vi "SWERVE_TRAJECTORY_READFILE_BEGIN.vi"(8 "ABS Odo Initialize":bool, 9 "Starting ChassisSpeeds":T4 {"vOmega" format="%10.3f"; "vY" format="%10.3f"; "vX" format="%10.3f"}, 10 "Write_Traj":bool=TRUE, 11 "Trajectory File Name":string="Sample-Robot-2-Trajectory-TrajLibrary.csv") -> (0 "error out":errorcluster, 1 "StartingPose":T1={"TRANSLATION"={"X"=0.0, "Y"=0.0}, "ROTATION"={"VALUE"=0.0, "COS"=1.0, "SIN"=0.0}} {"ROTATION"."SIN" format="%13.4f"; "ROTATION"."COS" format="%13.4f"; "ROTATION"."VALUE" format="%13.4f"; "TRANSLATION"."Y" format="%14.3f"; "TRANSLATION"."X" format="%14.3f"}, 2 "Trajectory Items":i32, 3 "TotalTImeSecs":dbl)   [LabVIEW 2023]
uses:
  <vilib>/Rock Robotics/WPI/ThirdParty/JAS_Junk/TrajLib/TypeDef/CHASSIS_SPEEDS.ctl
  <vilib>/Rock Robotics/WPI/ThirdParty/JAS_Junk/TrajLib/TypeDef/POSE2D.ctl
  <vilib>/Rock Robotics/WPI/ThirdParty/JAS_Junk/TrajLib/TypeDef/TRANSLATION2D.ctl
  <vilib>/Rock Robotics/WPI/ThirdParty/JAS_Junk/TrajLib/TypeDef/ROTATION2D.ctl
  <vilib>/Rock Robotics/WPI/ThirdParty/MJansen/PathPlanner/TypeDef/PathPlannerTrajectory.ctl
  <vilib>/Rock Robotics/WPI/ThirdParty/MJansen/PathPlanner/TypeDef/PathPlannerTrajectoryState.ctl
  <vilib>/Rock Robotics/WPI/ThirdParty/MJansen/PathPlanner/TypeDef/PathPlannerPathConstraints.ctl
  <vilib>/Rock Robotics/WPI/ThirdParty/MJansen/PathPlanner/TypeDef/PathPlannerPath.ctl
  <vilib>/Rock Robotics/WPI/ThirdParty/MJansen/PathPlanner/TypeDef/PathPlannerRotationTarget.ctl
  <vilib>/Rock Robotics/WPI/ThirdParty/MJansen/PathPlanner/TypeDef/PathPlannerConstraintsZone.ctl
  <vilib>/Rock Robotics/WPI/ThirdParty/MJansen/PathPlanner/TypeDef/PathPlannerEventMarker.ctl
  <vilib>/Rock Robotics/WPI/ThirdParty/MJansen/PathPlanner/TypeDef/PathPlannerCommandUtil.ctl
  <vilib>/Rock Robotics/WPI/ThirdParty/MJansen/PathPlanner/ENum/PathPlanner_CommandUtilType_ENUM.ctl
  <vilib>/Rock Robotics/WPI/ThirdParty/MJansen/PathPlanner/TypeDef/PathPlannerGoalEndState.ctl
  <vilib>/Rock Robotics/WPI/ThirdParty/MJansen/PathPlanner/TypeDef/PathPlannerPathPoint.ctl
  <vilib>/Rock Robotics/WPI/ThirdParty/MJansen/PathPlanner/VI/PathPlanner_Path_GetPoint.vi
  <vilib>/Rock Robotics/WPI/ThirdParty/JAS_Junk/TrajLib/Pose2d_New_TRRO.vi
  <vilib>/Rock Robotics/WPI/ThirdParty/MJansen/PathPlanner/VI/PathPlanner_PathPoint_GetAll.vi
  <vilib>/Rock Robotics/WPI/ThirdParty/JAS_Junk/TrajLib/Pose2d_getRotation.vi
  <vilib>/Rock Robotics/WPI/ThirdParty/JAS_Junk/TrajLib/Rotation2d_Minus.vi
  <vilib>/Rock Robotics/WPI/ThirdParty/JAS_Junk/TrajLib/VI/TimeInterpVariant_Clear.vi
  <vilib>/Rock Robotics/WPI/ThirdParty/JAS_Junk/TrajLib/Rotation2d_UnaryMinus.vi
  <vilib>/Rock Robotics/WPI/ThirdParty/JAS_Junk/TrajLib/Rotation2d_RotateBy.vi
  <vilib>/Rock Robotics/WPI/ThirdParty/JAS_Junk/TrajLib/Rotation2d_CreateXY.vi
  <vilib>/Rock Robotics/WPI/ThirdParty/JAS_Junk/TrajLib/Util_CalcDist.vi
  Swerve_Drive_System/SWERVE_DRIVE_GLOBALS.vi
  <vilib>/Rock Robotics/WPI/ThirdParty/JAS_Junk/TrajLib/Trajectory_Library.lvlib
  <vilib>/Rock Robotics/WPI/ThirdParty/MJansen/PathPlanner/PathPlanner24.lvlib
panel:
  # "Relative or absolute trajectory\nfile name"
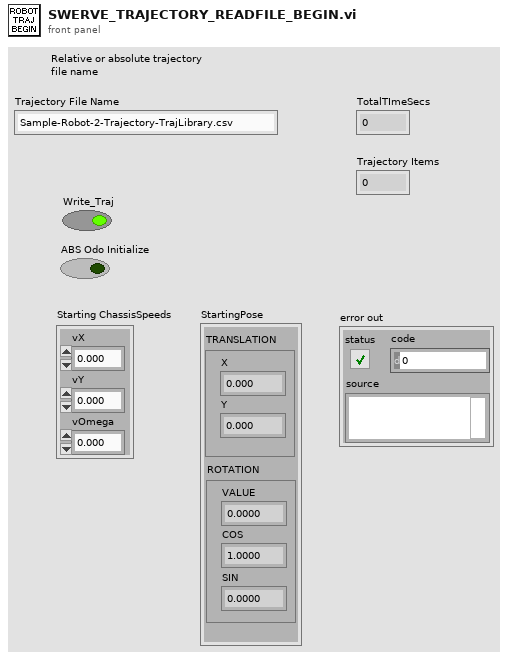
[diagram p1: front panel]
types:
  T1 = typedef "Trajectory_Library.lvlib/POSE2D.ctl" = cluster{"TRANSLATION":T2, "ROTATION":T3}
  T2 = typedef "Trajectory_Library.lvlib/TRANSLATION2D.ctl" = cluster{"X":dbl, "Y":dbl}
  T3 = typedef "Trajectory_Library.lvlib/ROTATION2D.ctl" = cluster{"VALUE":dbl, "COS":dbl, "SIN":dbl}
  T4 = typedef "Trajectory_Library.lvlib/CHASSIS_SPEEDS.ctl" = cluster{"vX":dbl, "vY":dbl, "vOmega":dbl}
  T5 = typedef "PathPlanner24.lvlib/PathPlannerPath.ctl" = cluster{"BezierPoints":T2[], "PreviewStartingRotation":T3, "Reversed":bool, "RotationTargets":T6[], "ConstraintZones":T7[], "EventMarkers":T9[], "GlobalConstraints":T8, "GoalEndState":T12, "AllPoints":T13[]}
  T6 = typedef "PathPlanner24.lvlib/PathPlannerRotationTarget.ctl" = cluster{"target":T3, "WaypointRelativePosition":dbl, "Exists":bool}
  T7 = typedef "PathPlanner24.lvlib/PathPlannerConstraintsZone.ctl" = cluster{"minWaypointPos":dbl, "maxWaypointPos":dbl, "Constraints":T8, "Present":bool}
  T8 = typedef "PathPlanner24.lvlib/PathPlannerPathConstraints.ctl" = cluster{"MaxVelocityMps;":dbl, "MaxAccelerationMpsSq;":dbl, "MaxAngularVelRadPsEc;":dbl, "MaxAngularAccRadPSecSq":dbl, "Exists":bool}
  T9 = typedef "PathPlanner24.lvlib/PathPlannerEventMarker.ctl" = cluster{"WaypointRelativePos":dbl, "minimumTriggerDistance":dbl, "markerPos":T2, "lastRobotPos":T2, "Command":T10, "markerPos Exists":bool, "LastRobotPoseExists":bool, "Triggered":bool}
  T10 = typedef "PathPlanner24.lvlib/PathPlannerCommandUtil.ctl" = cluster{"waitTime":dbl, "name":string, "pathName":string, "commands":cluster{"type":T11, "waitTime":dbl, "name":string, "pathName":string}[], "type":T11}
  T11 = typedef "PathPlanner24.lvlib/PathPlanner_CommandUtilType_ENUM.ctl" = enum16{"Unknown", "Wait", "Named", "Path", "Sequential", "Parallel", "Race", "Deadline"}
  T12 = typedef "PathPlanner24.lvlib/PathPlannerGoalEndState.ctl" = cluster{"Velocity":dbl, "Rotation":T3}
  T13 = typedef "PathPlanner24.lvlib/PathPlannerPathPoint.ctl" = cluster{"Position":T2, "HolonomicRotation":T3, "DistAlongPath":dbl, "CurveRadius":dbl, "MaxV":dbl, "Constraints":T8, "HolonomicRotationExists":bool}
  T14 = typedef "PathPlanner24.lvlib/PathPlannerTrajectory.ctl" = cluster{"States":T15[]}
  T15 = typedef "PathPlanner24.lvlib/PathPlannerTrajectoryState.ctl" = cluster{"TimeSeconds":dbl, "VelocityMPS":dbl, "AccerationMpsSq":dbl, "HeadingAngularVelRadPerSec":dbl, "PositionMeters":T2, "Heading":T3, "TargetHolonomicRotation":T3, "CurvatureRadPerMeter":dbl, "PathPlannerConstraints":T8, "DeltaPos":dbl}
  T16 = typedef "Trajectory_Library.lvlib/TRAJECTORY.ctl" = cluster{"TotalTImeSecs":dbl, "States":T17[]}
  T17 = typedef "Trajectory_Library.lvlib/TRAJ_STATE.ctl" = cluster{"TimeSeconds":dbl, "Velocity":dbl, "Acceleration":dbl, "POSE":T1, "Curvature":dbl}
  T18 = typedef "Trajectory_Library.lvlib/SWERVE_DRIVE_POSE_EST2.ctl" = cluster{"M_Vision_K":T19, "m_nominal_dT":dbl, "m_PrevTime_Sec":dbl, "Pose_Buffer":T20, "Swerve_Drive_Kinematics":T21, "Swerve_Drive_Odom":T23, "M_Q":T19, "NumModules":i32}
  T19 = typedef "NI_Matrix.lvlib/RealMatrix.ctl" = dbl[][]
  T20 = typedef "Trajectory_Library.lvlib/TIME_INTERPOLATABLE_VARIANT.ctl" = cluster{"TimeStamps":dbl[], "DataArray":variant[], "Min_TimeStamp":dbl, "Max_TimeStamp":dbl, "ItemCount":i32, "MaxBufferTime":dbl}
  T21 = typedef "Trajectory_Library.lvlib/SWERVE_DRIVE_KINEMATICS.ctl" = cluster{"NumModules":i32, "InverseKinematics":T19, "ForwardKinematics":T19, "Modules":T2[], "PrevCoR":T2, "SavedModuleStates":T22[]}
  T22 = typedef "Trajectory_Library.lvlib/SWERVE_DRIVE_MODULE_STATE.ctl" = cluster{"Speed":dbl, "Angle":T3}
  T23 = typedef "Trajectory_Library.lvlib/SWERVE_DRIVE_ODOMETRY.ctl" = cluster{"POSE":T1, "GyroOffset":T3, "PreviousAngle":T3, "PrevModulePositions":T24[], "NumModules":i32}
  T24 = typedef "Trajectory_Library.lvlib/SWERVE_DRIVE_MODULE_POSITION.ctl" = cluster{"Distance":dbl, "Angle":T3, "P":bool}
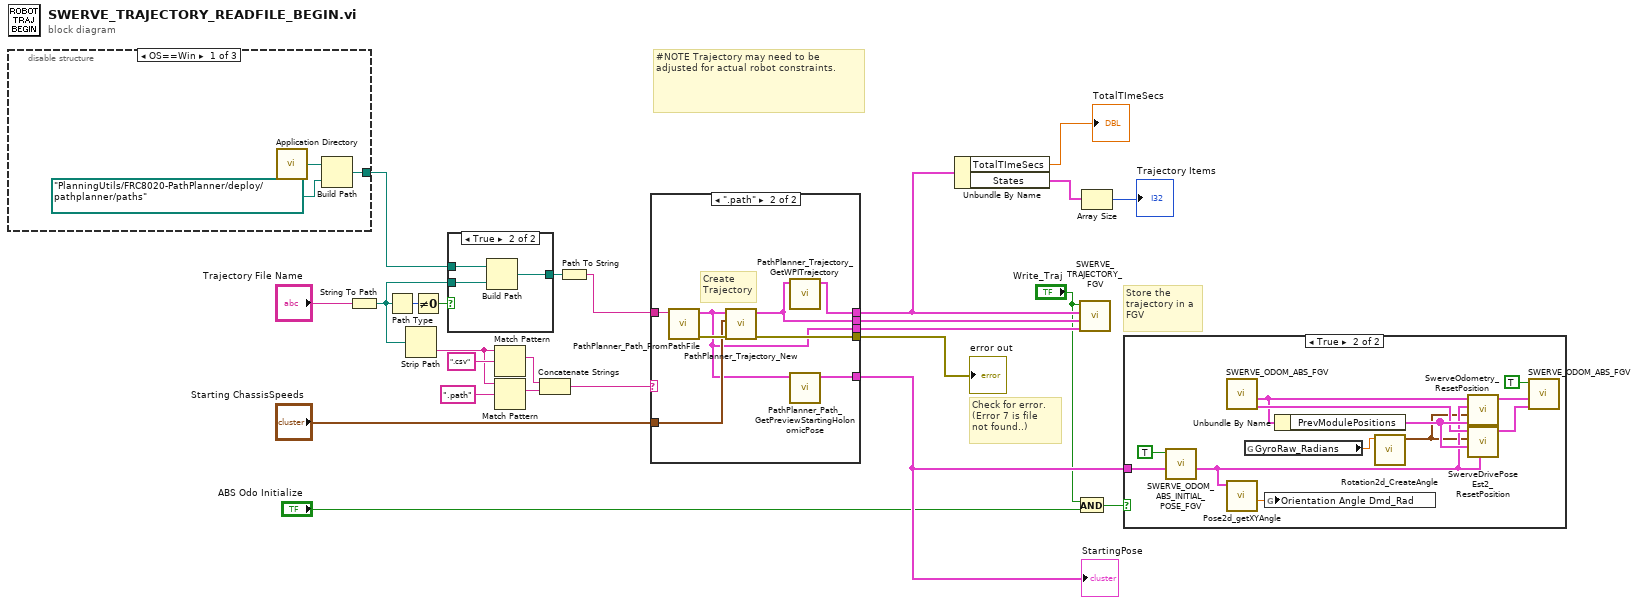
[diagram p0: block diagram]
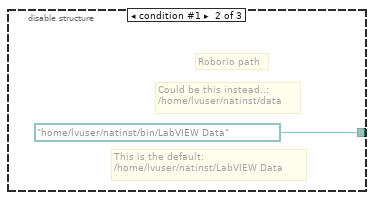
[diagram p2: hidden frame]
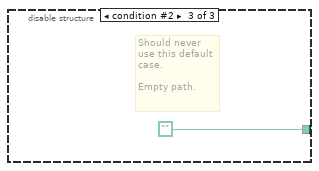
[diagram p3: hidden frame]
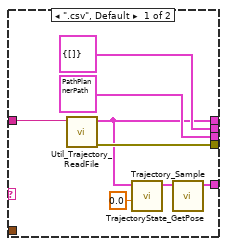
[diagram p5: hidden frame]
diagram:
  # "Check for error.  \n(Error 7 is file\nnot found..)"
  # "#NOTE Trajectory may need to be adjusted for actual robot constraints."
  # "Store the\ntrajectory in a \nFGV"
  n1 = disable-structure shown="OS==Win" {
    disable-tunnel: [w26 path "/home/lvuser/natinst/bin/LabVIEW Data" path ""] -> w18
    frame condition #0 (active) {
      n2 = call <vilib>:"Application Directory.vi"() -> ("Application Directory"=w28:path)
      n3 = Build Path(base path=w28, name or relative path=path "PlanningUtils/FRC8020-PathPlanner/deploy/pathplanner/paths") -> (appended path=w26:path)
    }
    frame condition #1 {
      # "This is the default:\n/home/lvuser/natinst/LabVIEW Data"
      # "Could be this instead..:\n/home/lvuser/natinst/data"
      # "Roborio path"
    }
    frame condition #2 {
      # "Should never\nuse this default\ncase.\n\nEmpty path."
    }
  }
  n4 = String To Path(string="Trajectory File Name") -> (path=w9:path)
  n5 = Path Type(1:w9) -> (0:w19:i16)
  n6 = Strip Path(path=w9) -> (name=w12:string)  [unwired: 1 out]
  n7 = Not Equal To 0?(x=w19) -> (x != 0?=w20:bool)
  n8 = case shown="True" w20 {
    tunnel: [w31 w34] -> w17
    tunnel: w18 -> [_ w33]
    tunnel: w9 -> [w31 w32]
    frame False {
    }
    frame True {
      n9 = Build Path(base path=w33, name or relative path=w32) -> (appended path=w34:path)
    }
  }
  n10 = Match Pattern(string=w12, regular expression=".csv") -> (match substring=w11:string)  [unwired: 1 in, 3 out]
  n11 = Match Pattern(string=w12, regular expression=".path") -> (match substring=w10:string)  [unwired: 1 in, 3 out]
  n12 = Concatenate Strings(w11, w10) -> (w8:string)
  n13 = Path To String(path=w17) -> (string=w15:string)
  n14 = case shown="\".path\"" w8 {
    tunnel: [w42 w48] -> w25
    tunnel: w15 -> [w41 w49]
    tunnel: [w36 w47] -> w7
    tunnel: "Starting ChassisSpeeds" -> [_ w46]
    tunnel: [T14 {"States"=[]} ("PathPlannerTrajectory") w45] -> w6
    tunnel: [T5 {"BezierPoints"=[], "PreviewStartingRotation"={"VALUE"=0.0, "COS"=1.0, "SIN"=0.0}, "Reversed"=FALSE, "RotationTargets"=[], "ConstraintZones"=[], "EventMarkers"=[], "GlobalConstraints"={"MaxVelocityMps;"=0.0, "MaxAccelerationMpsSq;"=0.0, "MaxAngularVelRadPsEc;"=0.0, "MaxAngularAccRadPSecSq"=0.0, "Exists"=FALSE}, "GoalEndState"={"Velocity"=0.0, "Rotation"={"VALUE"=0.0, "COS"=1.0, "SIN"=0.0}}, "AllPoints"=[]} ("PathPlannerPath") w44] -> w5
    tunnel: [w35 w43] -> w4
    frame ".csv", Default {
      n15 = call <vilib>:"Util_Trajectory_ReadFile.vi"("FileName"=w41) -> ("error out"=w42:errorcluster, "outTRAJECTORY"=w36:T16)  [unwired: 8 in, 1 out]
      n16 = call <vilib>:"Trajectory_Sample.vi"("Time"=0.0, "InputTRAJECTORY"=w36) -> ("OutputTRAJ_STATE"=w38:T17)  [unwired: 9 in]
      n17 = call <vilib>:"TrajectoryState_GetPose.vi"("TRAJ_STATE"=w38) -> ("TrajStatePose"=w35:T1)  [unwired: 10 in]
    }
    frame ".path" {
      # "Create\nTrajectory"
      n18 = call <vilib>:"PathPlanner_Path_FromPathFile.vi"("FileName"=w49) -> ("error out"=w48:errorcluster, "PathPlannerPath"=w44:T5)  [unwired: 8 in, 1 out]
      n19 = call <vilib>:"PathPlanner_Trajectory_New.vi"("StartingSpeeds"=w46, "Path"=w44) -> ("PathPlannerTrajectory"=w45:T14)  [unwired: 9 in]
      n20 = call <vilib>:"PathPlanner_Trajectory_GetWPITrajectory.vi"("PathPlannerTrajectory"=w45) -> ("WPI TRAJECTORY"=w47:T16)  [unwired: 9 in, 1 out]
      n21 = call <vilib>:"PathPlanner_Path_GetPreviewStartingHolonomicPose.vi"("PathPlannerPath"=w44) -> ("PreviewStartingPose"=w43:T1)  [unwired: 10 in]
    }
  }
  "error out" <- w25
  "StartingPose" <- w4
  n22 = Unbundle By Name(w7) -> ("TotalTImeSecs"=→"TotalTImeSecs":dbl, "States"=w23:T17[])
  n23 = And(x="Write_Traj", y="ABS Odo Initialize") -> (x .and. y?=w1:bool)
  n24 = call "SWERVE_TRAJECTORY_FGV.vi"("WRITE"="Write_Traj", "inTRAJECTORY"=w7, "inPathPlannerTrajectory"=w6, "inPathPlannerPath"=w5) -> ()  [unwired: 4 in, 3 out]
  n25 = Array Size(array=w23) -> (size(s)=→"Trajectory Items":i32)
  n26 = case shown="True" w1 {
    tunnel: w4 -> [_ w52]
    frame False {
    }
    frame True {
      n27 = call "SWERVE_ODOM_ABS_INITIAL_POSE_FGV.vi"("in INITIAL_POSE2D"=w52, "WRITE"=TRUE) -> ("out INITIAL_POSE2D"=w53:T1)  [unwired: 9 in]
      n28 = call "SWERVE_ODOM_ABS_FGV.vi"() -> ("out SWERVE_DRIVE_POSE_EST2"=w58:T18, "out SWERVE_DRIVE_ODOMETRY"=w56:T23)  [unwired: 10 in]
      n29 = call <vilib>:"Pose2d_getXYAngle.vi"("in POSE"=w53) -> ("Angle"=w55:dbl)  [unwired: 8 in, 2 out]
      n30 = global read "SWERVE_DRIVE_GLOBALS.vi" "GyroRaw_Radians"() -> (w50:dbl)
      n31 = global write "SWERVE_DRIVE_GLOBALS.vi" "Orientation Angle Dmd_Rad"(w55) -> ()
      n32 = Unbundle By Name(w56) -> ("PrevModulePositions"=w59:T24[])
      n33 = call <vilib>:"Rotation2d_CreateAngle.vi"("Angle"=w50) -> ("ROTATION"=w51:T3)  [unwired: 10 in]
      n34 = call <vilib>:"SwerveOdometry_ResetPosition.vi"("Module Positions"=w59, "gyroAngle"=w51, "Pose"=w53, "in SWERVE_DRIVE_ODOMETRY"=w56) -> ("out SWERVE_DRIVE_ODOMETRY"=w60:T23)  [unwired: 6 in, 1 out]
      n35 = call <vilib>:"SwerveDrivePoseEst2_ResetPosition.vi"("Pose"=w53, "Module Positions"=w59, "Gyro"=w51, "in SwerveDrivePoseEst2"=w58) -> ("Out SwerveDrivePoseEst2"=w61:T18)  [unwired: 7 in]
      n36 = call "SWERVE_ODOM_ABS_FGV.vi"("in SWERVE_DRIVE_POSE_EST2"=w61, "in SWERVE_DRIVE_ODOMETRY"=w60, "WRITE"=TRUE) -> ()  [unwired: 7 in, 2 out]
    }
  }
